vi "Monitor OPC Items with DataSocket.vi"() -> ()   [LabVIEW 2023]
doc: "This VI uses the DataSocket functions to read values from an OPC server. You can specify which URL you want to read. The National Instruments.OPCDemo server provides the possible OPC URLs for this example."
panel:
  out "Selected URL":string
  out "OPC Data":dbl(graph)
  in  "Stop":bool
  # "Overview: Demonstrates the use of the DataSocket functions to read data from an OPC server.\nRequirements: Windows, LabVIEW 32-bit\nInstructions:\n1. Run the VI. Note: If you run this example in LabVIEW 64-bit, it will return an error.\n2. In the dialog that appears, select one of the demo OPC URLs under the Computer > National Instruments.OPCDemo > NI OPC Demo Server > Function Items category and click OK.\n3. The OPC Data chart will begin updating with values from the specified OPC URL.\n4. Click Stop to stop the VI."
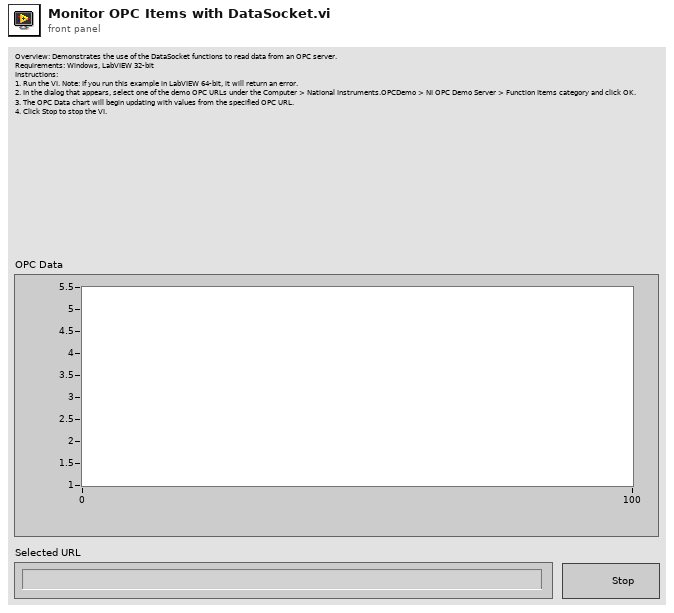
[diagram p1: front panel]
types:
  T1 = enum16{"Read", "Write", "ReadWrite", "BufferedRead", "BufferedReadWrite"}
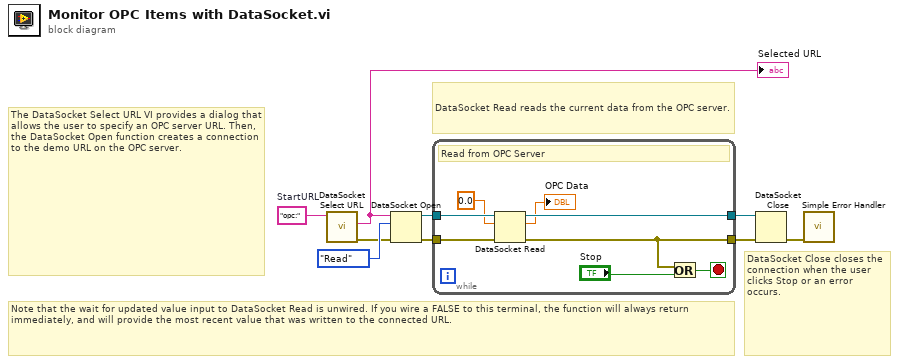
[diagram p0: block diagram]
diagram:
  w4 = "opc:"  # StartURL
  # "Note that the wait for updated value input to DataSocket Read is unwired. If you wire a FALSE to this terminal, the function will always return immediately, and will provide the most recent value that was written to the connected URL."
  # "The DataSocket Select URL VI provides a dialog that allows the user to specify an OPC server URL. Then, the DataSocket Open function creates a connection to the demo URL on the OPC server."
  # "DataSocket Close closes the connection when the user clicks Stop or an error occurs."
  # "DataSocket Read reads the current data from the OPC server."
  n1 = call <vilib>:"DataSocket Select URL.vi"("StartURL (empty)"=w4) -> ("error out"=w2:errorcluster, "URL"=w1:string)  [unwired: 2 in, 7 out]
  "Selected URL" <- w1
  n2 = DataSocket Open(8:w2, 10:T1."Read" ("mode"), 11:w1) -> (0:w7:errorcluster, 3:w9:refnum<k13>)  [unwired: 1 out]
  n3 = while {
    tunnel: [w11] -> w6
    tunnel: w7 -> [w15]
    tunnel: [w16] -> w8
    tunnel: w9 -> [w17]
    stop <- w14 stop-if-true
    # "Read from OPC Server"
    n4 = DataSocket Read(8:w15, 10:0.0, 11:w17) -> (0:w11:errorcluster, 2:→"OPC Data":dbl, 3:w16:refnum<k13>)  [unwired: 6 out]
    n5 = Or(x=w11, y="Stop") -> (x .or. y?=w14:bool)
  }
  n6 = DataSocket Close(8:w6, 11:w8) -> (0:w3:errorcluster)  [unwired: 2 out]
  n7 = call <vilib>:"Simple Error Handler.vi"("error in (no error)"=w3) -> ()  [unwired: 4 in, 5 out]
